vi "3-1 controllo se compreso IF AND (ex 2-1 control) facile ris control.vi"(1 "control":bool, 2 "low limit":dbl(knob) scale=0.0..10.0 scale format="%.1f", 3 "high limit":dbl(knob) scale=0.0..10.0 scale format="%.1f", 4 "data in":dbl format="%.2f") -> (0 "data out":dbl(knob) scale=0.0..10.0 scale format="%.1f")   [LabVIEW 2012]
panel:
  # "Se control = ON, bisogna verificare che il valore sia compreso nei limiti\n                     trasferendo il valore di ingresso diviso per il range ( high limit-low limit)\n                     in uscita se ci˜ si verifica; in caso contrario o \nse control = OFF, non viene effettuato nessun controllo e il valore di ingresso passa\n                    direttamente in uscita"
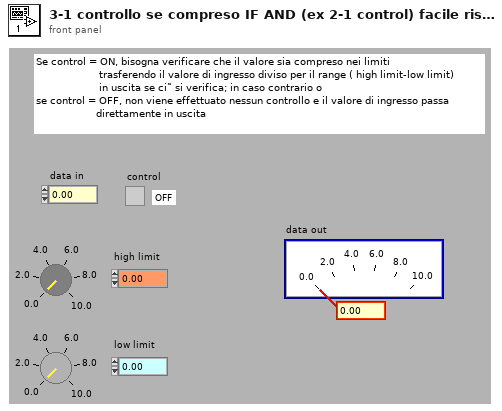
[diagram p1: front panel]
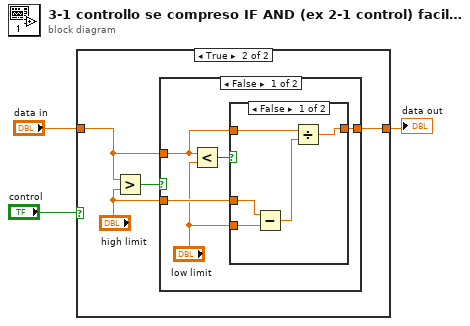
[diagram p0: block diagram]
diagram:
  n1 = case shown="True" "control" {
    tunnel: "data in" -> [w4 w7]
    tunnel: [w4 w6] -> w1
    frame False {
    }
    frame True {
      n2 = Greater?(x=w7, y="high limit") -> (0:w8:bool)
      n3 = case shown="False" w8 {
        tunnel: w7 -> [w12 w20]
        tunnel: [w11 w20] -> w6
        tunnel: "high limit" -> [w10 _]
        frame False {
          n4 = Less?(x=w12, y="low limit") -> (x < y?=w13:bool)
          n5 = case shown="False" w13 {
            tunnel: w12 -> [w15 w19]
            tunnel: [w14 w19] -> w11
            tunnel: w10 -> [w17 _]
            tunnel: "low limit" -> [w16 _]
            frame False {
              n6 = Subtract(x=w17, y=w16) -> (x-y=w18:dbl)
              n7 = Divide(x=w15, y=w18) -> (x/y=w14:dbl)
            }
            frame True {
            }
          }
        }
        frame True {
        }
      }
    }
  }
  "data out" <- w1
